vi "Array in place.vi"   [LabVIEW 2013, in "NISE Tools Drop Templates.lvlib"]
uses:
  NISE Tools Drop Templates.lvlib
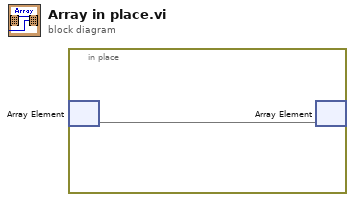
[diagram p0: block diagram]
diagram:
  n1 = in-place {
    n2 = in-place-array #1() -> (w1)  [unwired: 2 in]
    n3 = in-place-array #1(w1) -> ()  [unwired: 2 out]
  }
